vi "Transmit Reference (FPGA).vi"() -> ()   [LabVIEW 2019]
uses:
  SubVIs/Tone Generator/Channel Control.ctl
  SubVIs/Sync/Sync Control.ctl
  SubVIs/Sync/Sync Measurements.ctl
  <instrlib>/_niInstr/DSP/v1/Shared/Public/IQ Impairments.ctl
  <instrlib>/_niInstr/DSP/v1/Shared/Public/Filter Coefficients.ctl
  Host/SubVIs/Low-level/TypeDefs/Gain Setting.ctl
  <instrlib>/niMmWave/ni3620/Config/v1/FPGA/Public/Typedefs/TX1 RX1 Port.ctl
  <vilib>/Platform/TimedLoop/XDataNode/timing_clust.ctl
  <vilib>/Platform/TimedLoop/XDataNode/nitl_modes.ctl
  <vilib>/Platform/TimedLoop/XDataNode/wakeup.ctl
  <instrlib>/_niInstr/DSP/v1/Shared/Public/IQ Data.ctl
  <vilib>/rvi/Emulation/niFpgaSctlEmulationGetInTimedLoop.vi
  <vilib>/rvi/Emulation/niFpgaEmulationReportErrorSimple.vi
  <vilib>/rvi/Emulation/niFpgaGetClockAttributes.vi
  <vilib>/rvi/Emulation/niFpgaCriticalErrorInLSC.vi
  <vilib>/rvi/Emulation/niFpgaProcessEmulError.vi
  <vilib>/rvi/eio/common/nirviEmuTemplateMethod_errors.vi
  SubVIs/Misc/Globals.vi
  <vilib>/rvi/interface/RandomDataEmulation/nirviRandomDataMultiElementFPGAFIFO.vi
  <instcachedir>/0/nirviRandomDataMultiElementFPGAFIFO_1ED88BA00AC641F388A9B1FAA20E354D.lvgen/nirviRandomDataMultiElementFPGAFIFO_1ED88BA00AC641F388A9B1FAA20E354D_003.vi
  <vilib>/rvi/interface/RandomDataEmulation/niFpgaRandomDataHandleErrors.vi
  <instrlib>/_niInstr/Basic Elements/v1/FPGA/Private/Count Up U16.vi
  <instrlib>/_niInstr/Data Formatting/v1/FPGA/Private/Convert/U32 array to Boolean Array.vi
  <vilib>/rvi/Memory/Memory_Emulation/nirvimemoryFastEmulation.vi
  <vilib>/rvi/Memory/Memory_Emulation/nirvimemoryEmulation.vi
  <vilib>/rvi/Emulation/niFpgaEmulationIsFPGAContextNoSignature.vi
  <vilib>/rvi/DataTransferAndStorage/Container/Common/niFpgaContainerGetUniqueNameForEmu.vi
  <vilib>/rvi/errors/nirviReportUnexpectedCaseInternalError (U32).vi
  <instrlib>/_niInstr/Data Formatting/v1/FPGA/Private/Convert/U8 array to Boolean Array.vi
  <instrlib>/_niInstr/Data Formatting/v1/FPGA/Private/Convert/Boolean Array to U32 Array.vi
  <vilib>/rvi/errors/niFpgaSetErrorForExecOnDevCompSimple.vi
  <vilib>/rvi/eio/common/nirviEmuReportErrorAndStop.vi
  <vilib>/rvi/FIFO/Fifo_Resource/nirvififoEmulationSetSize.vi
  <vilib>/rvi/FIFO/Fifo_Resource/nirviFifoEmulationQueueMgr.vi
  <instcachedir>/0/nirviFifoEmulationQueueMgr_E5CAEC123FF24DC58D834DCA3CDAA9B5.lvgen/nirviFifoEmulationQueueMgr_E5CAEC123FF24DC58D834DCA3CDAA9B5_008.vi
  <vilib>/rvi/FIFO/Fifo_Resource/nirvififoEmulationDetermineInputValidOut.vi
  <vilib>/rvi/FIFO/Fifo_Resource/nirvififoEmulationCreateLock.vi
  <vilib>/rvi/FIFO/Fifo_Resource/nirvififoEmulationObtainLock.vi
  <vilib>/rvi/FIFO/Fifo_Resource/nirvififoEmulationReleaseLock.vi
  <vilib>/rvi/occurrence/nirviWaitOnOccurrenceBase.vi
  <vilib>/rvi/errors/nirviReportUnexpectedCaseInternalError.vi
  <instrlib>/_niInstr/Basic Elements/v1/FPGA/Private/Count Up U8.vi
  <vilib>/rvi/DataTransferAndStorage/Container/Common/niFpgaContainerSetEmuInfo.vi
  <vilib>/Utility/error.llb/Clear Errors.vi
  <vilib>/Platform/TimedLoop/XDataNode/XDataNode.xnode
  <vilib>/eio/EIONode/EIONode.xnode
  <vilib>/eio/EIOMethodNode/EIOMethodNode.xnode
  <vilib>/rvi/DataTransferAndStorage/Container/XNode/niFpgaContainer.xnode
  <vilib>/rvi/interface/RandomDataEmulation/nirviRandomDataFpgaMultiElementTemplate.vi
  <vilib>/rvi/FIFO/Fifo_Resource/nirvififoEmulationWrite.vi
  <vilib>/rvi/LocalResourceManager/LocalResourceManager.xnode
  <vilib>/rvi/FIFO/Fifo_Resource/nirvififoEmulationRead.vi
  <vilib>/Platform/TimedLoop/XDataNode/XDNodeRunTimeDep.lvlib
  <instrlib>/_niInstr/Basic Elements/v1/FPGA/niInstr Basic Elements v1 FPGA.lvlib
  <instrlib>/_niInstr/Data Formatting/v1/FPGA/niInstr Data Formatting v1 FPGA.lvlib
  <instrlib>/_niInstr/DSP/v1/Shared/niInstr DSP v1 Shared.lvlib
  <instrlib>/niMmWave/ni3620/Config/v1/FPGA/niMmWave Config v1 FPGA.lvlib
panel:
  in  "sync.master reset listen":bool
  in  "sync.counter reset enable":bool
  in  "20 kHz tclk parameters":T1
  out "sysref value":u8
  out "tclk value":u16
  in  "gain ranging.enable port config":bool
  in  "gain ranging.enable coarse gain ranging":bool
  in  "gain ranging.enable fine gain ranging":bool
  in  "gain ranging.coarse gain values":fxp<+/-,16,12>[](array[numeric])=[0.0, 0.0, 0.0, 0.0]
  out "port 5.debug info":T2
  out "port 5.rx fifo overflow":bool
  in  "port 5.rx fifo overflow clear":bool
  out "port 4.rx fifo overflow":bool
  in  "port 4.rx fifo overflow clear":bool
  out "port 4.debug info":T2
  out "aurora.fifo 1 overflow":bool
  in  "aurora.reset trigger":bool
  out "aurora.fifo 0 overflow":bool
  in  "aurora.fifo overflow clear":bool
  in  "aurora.write":bool
  out "clocks valid":bool[](array[boolean])
  in  "table info":T3
  in  "gain ranging.manual setting":T6
  in  "gain ranging.setting list step":T7
  in  "gain ranging.enable":bool
  in  "gain ranging.dwell time (cycles)":u32=4800
  in  "txjesd.control":T8
  out "txjesd.status":T9
  in  "filter.enable":bool
  in  "filter.coefficients":T10
  in  "cal.correction":T12={"sample delay"={"I delay"=0.0, "Q delay"=0.0}, "fractional delay"={"enable"=FALSE, "coef write"=FALSE, "coef data"=0.0}, "impairments"={"inline gain I"=0.9999923706054688, "inline gain Q"=0.9999923706054688, "cross gain I"=0.0, "cross gain Q"=0.0, "pre-gain offset I"=0.0, "pre-gain offset Q"=0.0, "post-gain offset I"=0.0, "post-gain offset Q"=0.0}, "iq inversion"={"invert I"=FALSE, "invert Q"=FALSE}}
  out "sync.measurements":T13
  in  "sync.parameters":T15
  in  "sync.use synced trigger":bool
  in  "sync.trigger":bool
  in  "gen.read":bool
  in  "cal.generation":T16={"generation select"=enum."Pass Through", "tone parameters"={"frequency"=0.125, "gain"=0.5}, "pulse parameters"={"frequency"=16, "gain"=0.5, "width"=16}}
  in  "gen.load":bool
  in  "gen.triggered read":bool
  in  "gen.length":u16=15
  in  "gen.write enable":bool
  in  "tone.routing":cluster{"I":T17, "Q":T17}
  in  "tone.parameters":T18(array[cluster])=[{"frequency"=0.032551999999999026, "gain"=0.8000030517578125, "phase"=0.0, "offset"={"offset I"=0.0, "offset Q"=0.0}}, {"frequency"=0.032551999999999026, "gain"=0.0, "phase"=0.0, "offset"={"offset I"=0.0, "offset Q"=0.0}}] {"offset"."offset Q" format="%#.18g"; "offset"."offset I" format="%#.18g"}
  in  "waveform type":enum16{"Tone", "Waveform Generation"}(ring)
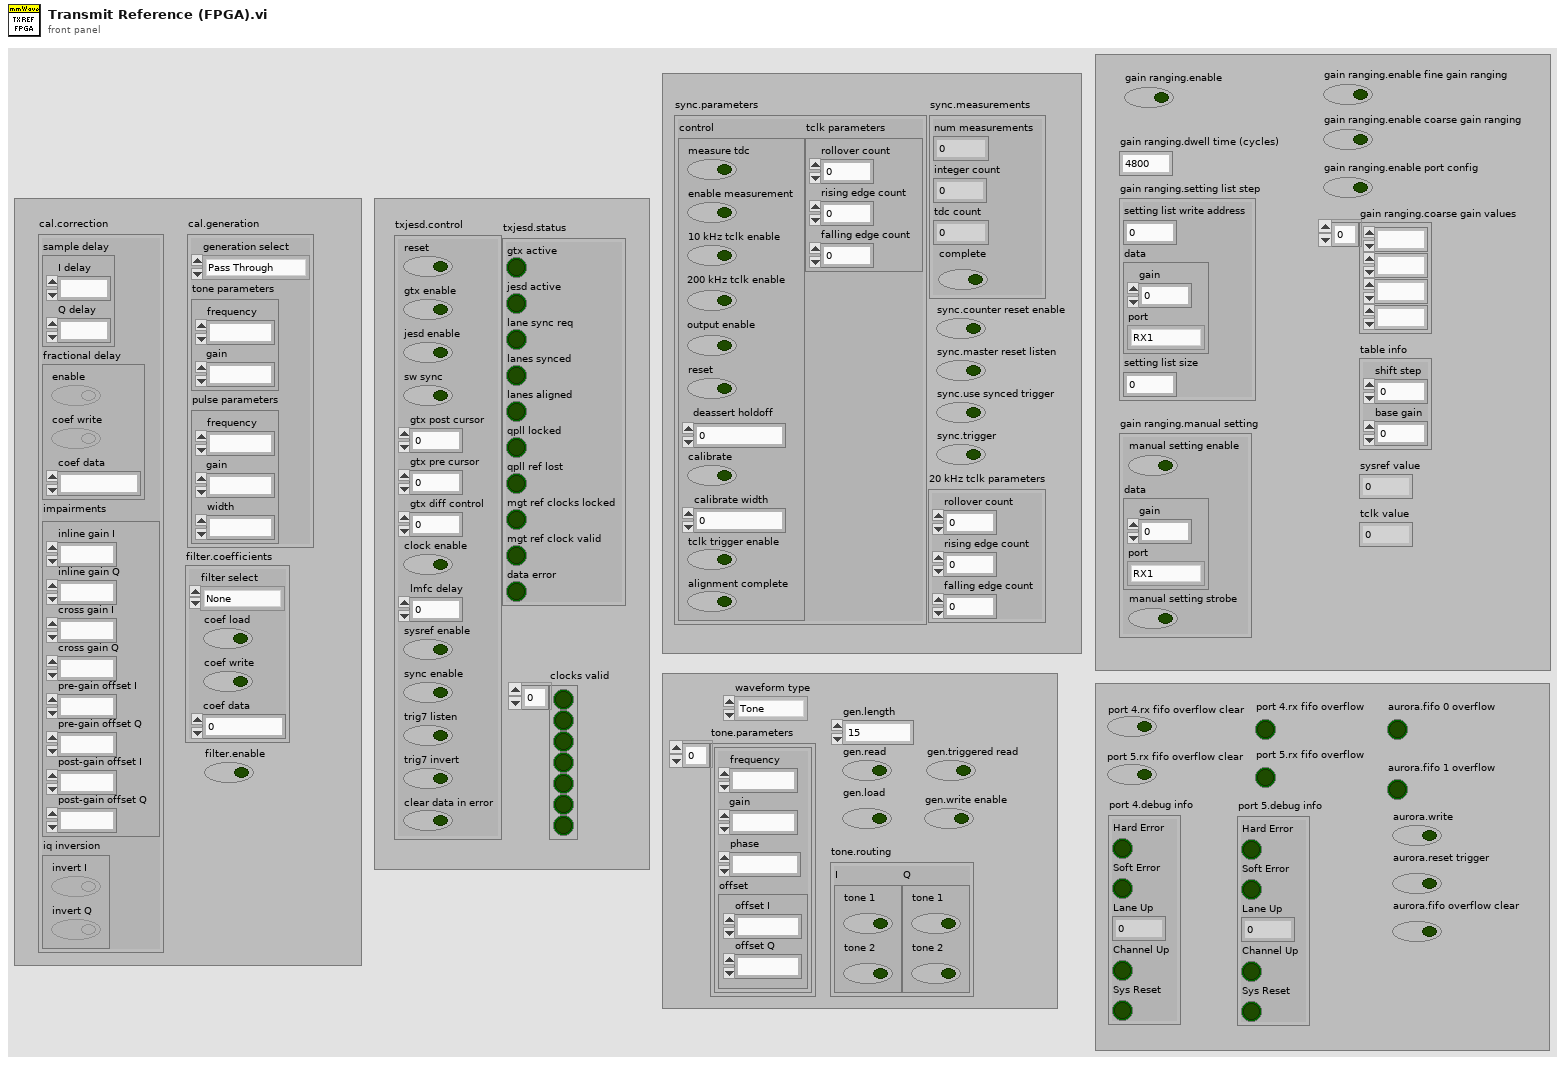
[diagram p1: front panel]
types:
  T1 = cluster{"rollover count":u16, "rising edge count":u16, "falling edge count":u16}
  T2 = cluster{"Hard Error":bool, "Soft Error":bool, "Lane Up":fxp<+,4,4>, "Channel Up":bool, "Sys Reset":bool}
  T3 = cluster{"shift step":i16, "base gain":fxp<+/-,16,12>}
  T4 = typedef "gain setting.ctl" = cluster{"gain":fxp<+/-,16,12>, "port":T5}
  T5 = typedef "TX1 RX1 Port.ctl" = enum8{"RX1", "TX1/RX2"}
  T6 = cluster{"manual setting enable":bool, "data":T4, "manual setting strobe":bool}
  T7 = cluster{"setting list write address":u32, "data":T4, "setting list size":u16}
  T8 = cluster{"reset":bool, "gtx enable":bool, "jesd enable":bool, "sw sync":bool, "gtx post cursor":fxp<+,5,5>, "gtx pre cursor":fxp<+,5,5>, "gtx diff control":fxp<+,4,4>, "clock enable":bool, "lmfc delay":fxp<+,5,5>, "sysref enable":bool, "sync enable":bool, "trig7 listen":bool, "trig7 invert":bool, "clear data in error":bool}
  T9 = cluster{"gtx active":bool, "jesd active":bool, "lane sync req":bool, "lanes synced":bool, "lanes aligned":bool, "qpll locked":bool, "qpll ref lost":bool, "mgt ref clocks locked":bool, "mgt ref clock valid":bool, "data error":bool}
  T10 = typedef "niInstr DSP v1 Shared.lvlib/Filter Coefficients.ctl" = cluster{"filter select":enum8{"None", "I Inline", "I Cross", "Q Cross", "Q Inline"}, "coef load":bool, "coef write":bool, "coef data":fxp<+/-,18,1>}
  T11 = typedef "niInstr DSP v1 Shared.lvlib/IQ Impairments.ctl" = cluster{"inline gain I":fxp<+/-,18,1>, "inline gain Q":fxp<+/-,18,1>, "cross gain I":fxp<+/-,18,1>, "cross gain Q":fxp<+/-,18,1>, "pre-gain offset I":fxp<+/-,18,1>, "pre-gain offset Q":fxp<+/-,18,1>, "post-gain offset I":fxp<+/-,18,1>, "post-gain offset Q":fxp<+/-,18,1>}
  T12 = cluster{"sample delay":cluster{"I delay":fxp<+,13,13>, "Q delay":fxp<+,13,13>}, "fractional delay":cluster{"enable":bool, "coef write":bool, "coef data":fxp<+/-,18,1>}, "impairments":T11, "iq inversion":cluster{"invert I":bool, "invert Q":bool}}
  T13 = typedef "Sync Measurements.ctl" = cluster{"num measurements":u16, "integer count":u16, "tdc count":u16, "complete":bool}
  T14 = typedef "Sync Control.ctl" = cluster{"measure tdc":bool, "enable measurement":bool, "10 kHz tclk enable":bool, "200 kHz tclk enable":bool, "output enable":bool, "reset":bool, "deassert holdoff":u8, "calibrate":bool, "calibrate width":u8, "tclk trigger enable":bool, "alignment complete":bool}
  T15 = cluster{"control":T14, "tclk parameters":cluster{"rollover count":u16, "rising edge count":u16, "falling edge count":u16}}
  T16 = cluster{"generation select":enum16{"Pass Through", "Tone", "Pulse", "Disable"}, "tone parameters":cluster{"frequency":fxp<+/-,48,0>, "gain":fxp<+/-,18,1>}, "pulse parameters":cluster{"frequency":u32, "gain":fxp<+/-,18,1>, "width":u8}}
  T17 = typedef "Channel Control.ctl" = cluster{"tone 1":bool, "tone 2":bool}
  T18 = cluster{"frequency":fxp<+/-,48,0>, "gain":fxp<+/-,18,1>, "phase":fxp<+/-,21,0>, "offset":cluster{"offset I":fxp<+/-,18,1>, "offset Q":fxp<+/-,18,1>}}[]
  T19 = cluster{"s_axis_tvalid":refnum<k21>, "s_axis_tdata_0":refnum<k21>, "s_axis_tdata_1":refnum<k21>, "s_axis_tdata_2":refnum<k21>, "s_axis_tdata_3":refnum<k21>, "s_axis_tready":refnum<k21>}
  T20 = cluster{"m_axis_tvalid":refnum<k21>, "m_axis_tdata_0":refnum<k21>, "m_axis_tdata_1":refnum<k21>, "m_axis_tdata_2":refnum<k21>, "m_axis_tdata_3":refnum<k21>}
  T21 = typedef "Sync Resources.ctl" = cluster{"tdc assert":refnum<k21>, "tdc deassert":refnum<k21>, "tdc count":refnum<k21>, "control":refnum<k21>, "integer count":refnum<k21>}
  T22 = typedef "XDNodeRunTimeDep.lvlib/timing_clust.ctl" = cluster{"Expected End [f-1]":u64, "Actual End [f-1]":u64, "Finished Late? [f-1]":bool, "Expected End [i-1]":u64, "Actual End [i-1]":u64, "Finished Late? [i-1]":bool, "Expected Start [i]":u64, "Actual Start [i]":u64, "Expected Start [f]":u64, "Actual Start [f]":u64, "Source Name":string, "Structure Name":string, "Period":i64, "Deadline":i64, "Offset":i64, "Start":i64, "Priority":i32, "Timeout":i32, "Mode":T23, "Wakeup Reason":T24, "Error":errorcluster, "Source Type":string, "Secondary Source Type":string, "Global End Time":u64, "Global Start Time":u64, "Frame Duration":u64, "Iteration Duration":u64, "Assigned CPU":i32, "I/O Scan Engine Mode":u32}
  T23 = typedef "XDNodeRunTimeDep.lvlib/nitl_modes.ctl" = enum32{"No Change", "Process missed periods, maintain original phase", "Discard missed periods, maintain original phase", "Process missed periods, ignore original phase", "Discard missed periods, ignore original phase"}
  T24 = typedef "XDNodeRunTimeDep.lvlib/wakeup.ctl" = enum32{"Normal", "Aborted", "Asynchronous wakeup", "Timing source error", "Timed loop error", "Timeout"}
  T25 = typedef "AXI4-Stream Reader FXP64x4 Resources.ctl" = cluster{"AXI4-Stream Reader Resources":cluster{"Use TREADY":bool, "Use TLAST":bool, "TLAST":refnum<k21>, "TREADY":refnum<k21>, "TVALID":refnum<k21>, "Use TKEEP":bool, "Use TSTRB":bool, "Use TUSER":bool}, "TDATA Resources":cluster{"TDATA_0":refnum<k21>, "TDATA_1":refnum<k21>, "TDATA_2":refnum<k21>, "TDATA_3":refnum<k21>}, "TKEEP":refnum<k21>, "TSTRB":refnum<k21>}
  T26 = typedef "AXI4-Stream Writer FXP64x4 Resources.ctl" = cluster{"Writer Resources":cluster{"Use TREADY":bool, "Use TLAST":bool, "TLAST":refnum<k21>, "TREADY":refnum<k21>, "TVALID":refnum<k21>, "Use TSTRB":bool, "Use TKEEP":bool, "Use TUSER":bool}, "TDATA Resources":cluster{"TDATA_0":refnum<k21>, "TDATA_1":refnum<k21>, "TDATA_2":refnum<k21>, "TDATA_3":refnum<k21>}, "TKEEP":refnum<k21>, "TSTRB":refnum<k21>}
  T27 = cluster{"disable TClk measure":bool, "output enable":bool, "output value":bool}
  T28 = typedef "niInstr DSP v1 Shared.lvlib/IQ Data.ctl" = cluster{"I":fxp<+/-,18,1>, "Q":fxp<+/-,18,1>, "overflow":bool}
  T29 = cluster{"Hard Error":refnum<k21>, "Soft Error":refnum<k21>, "Lane Up":refnum<k21>, "Channel Up":refnum<k21>, "Sys Reset":refnum<k21>}
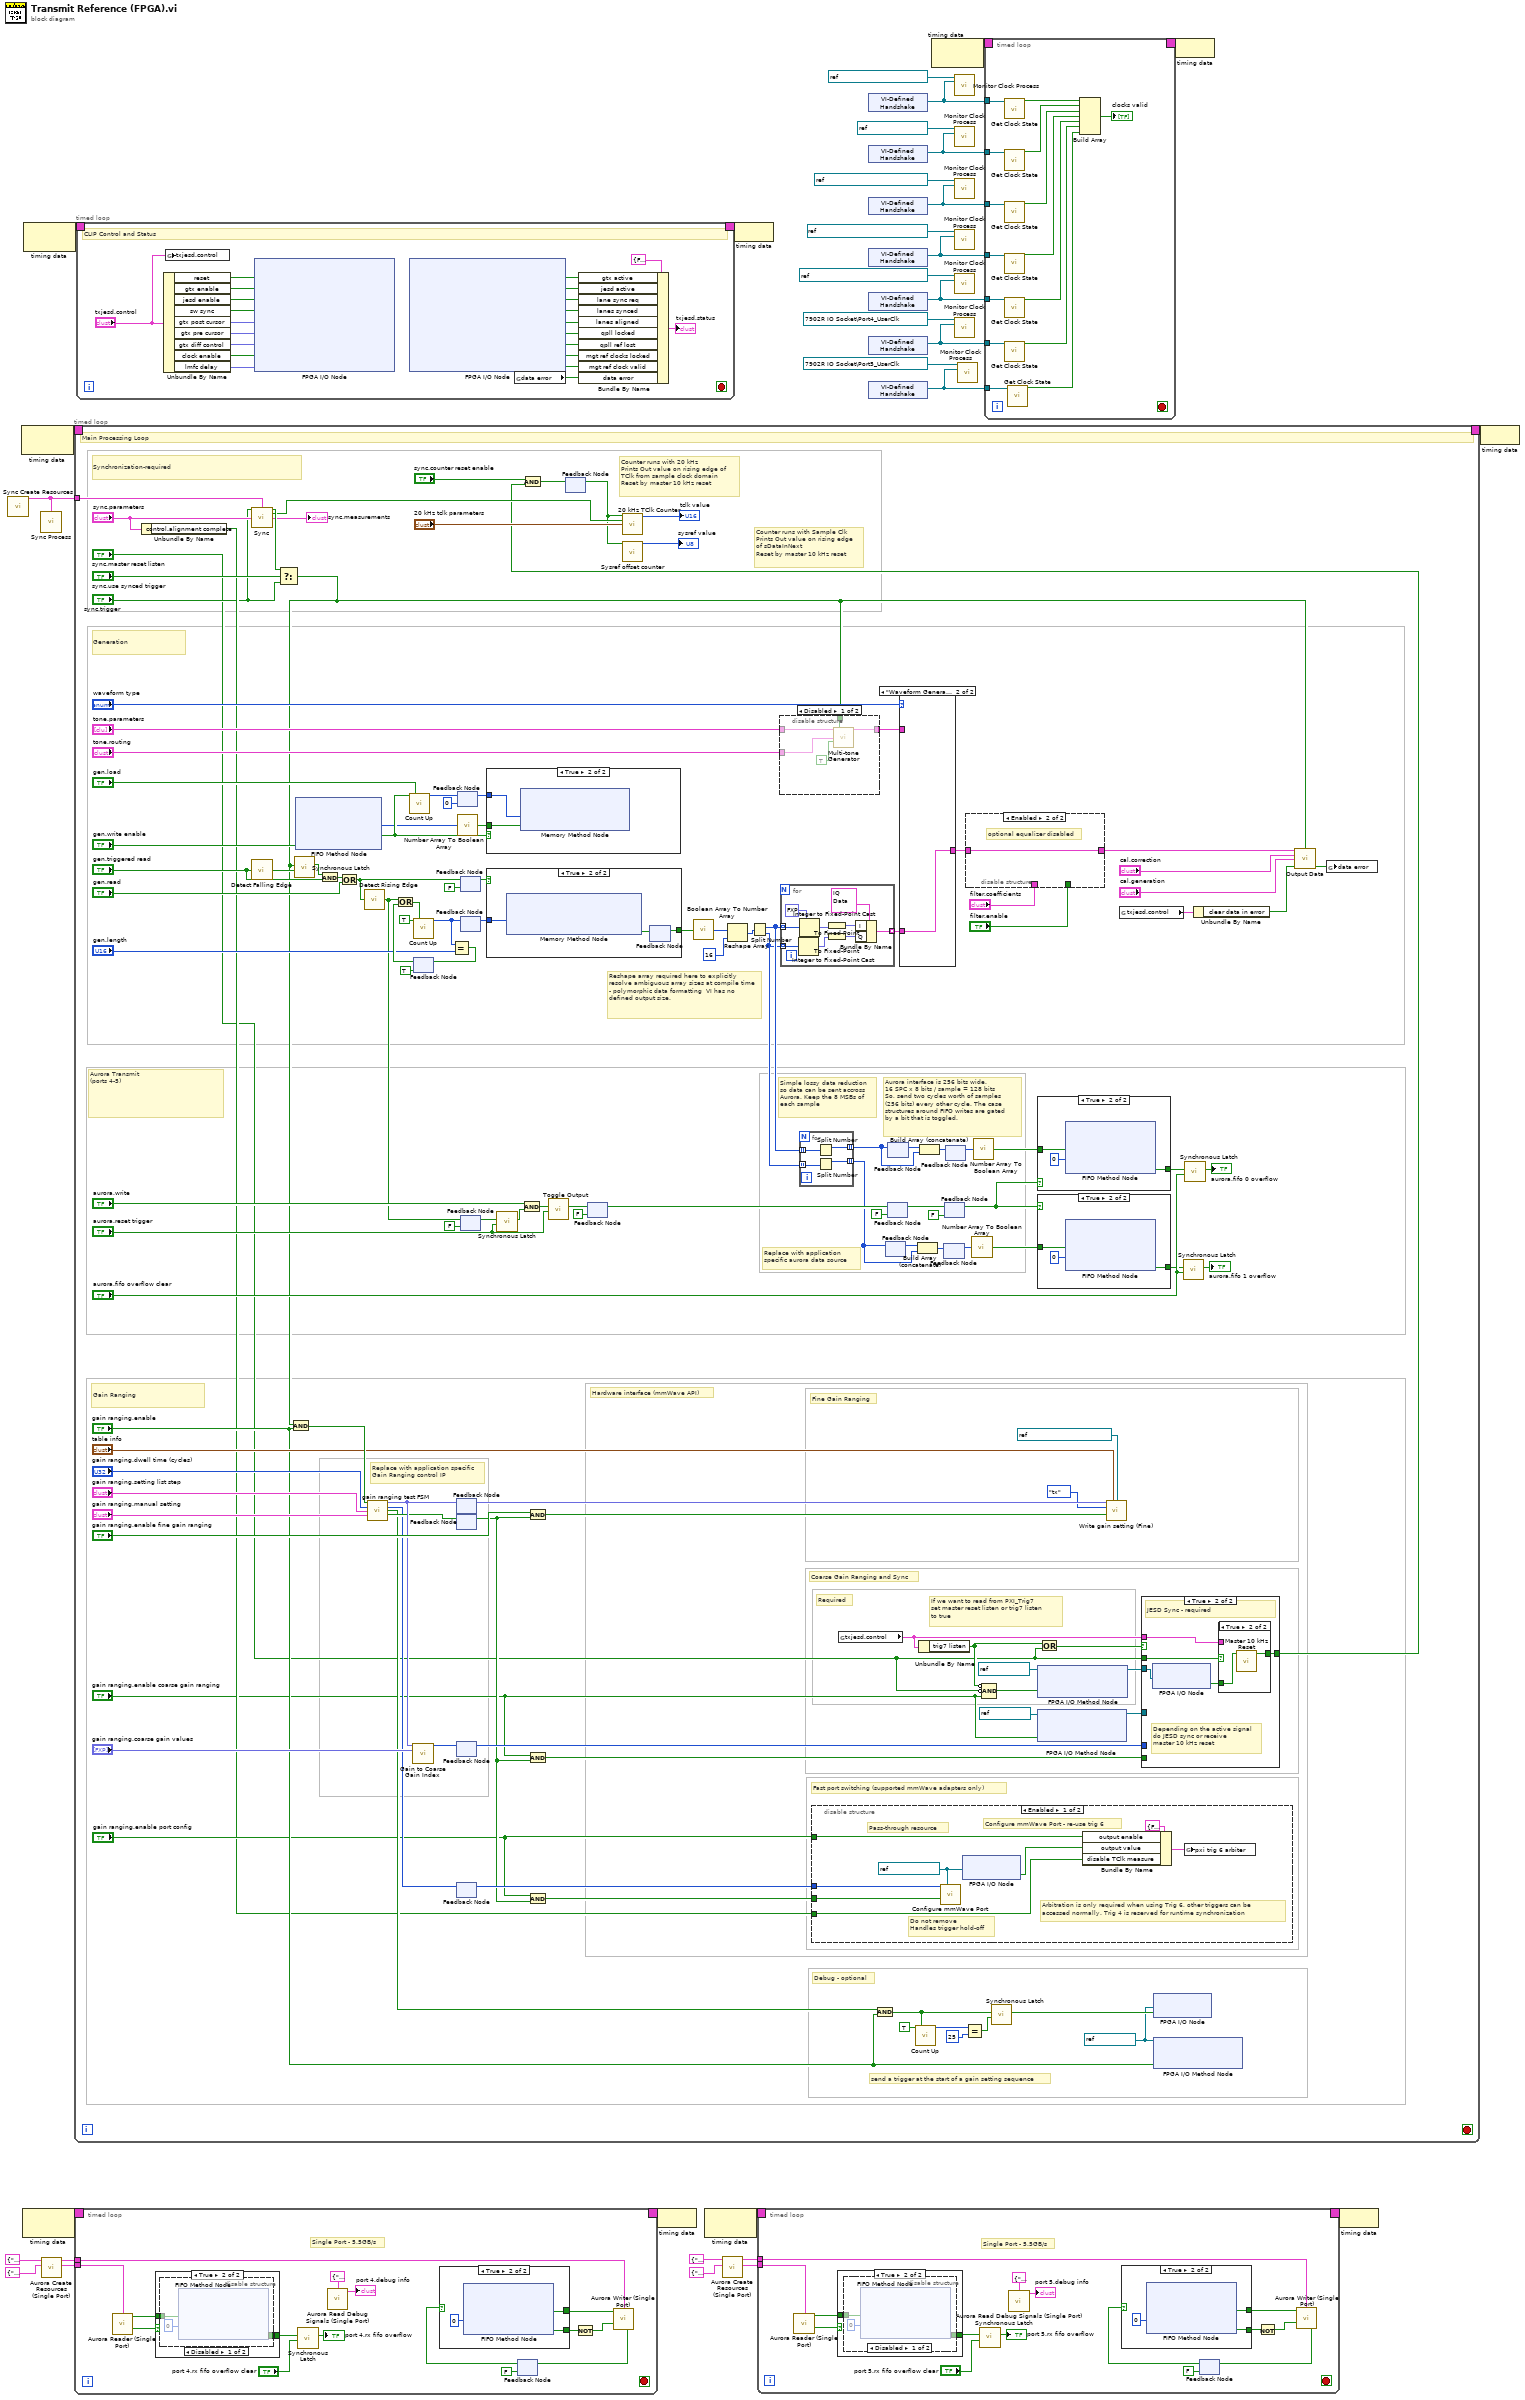
[diagram p0: block diagram]
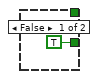
[diagram p2: hidden frame]
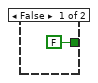
[diagram p3: hidden frame]
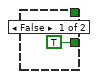
[diagram p5: hidden frame]
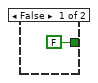
[diagram p6: hidden frame]
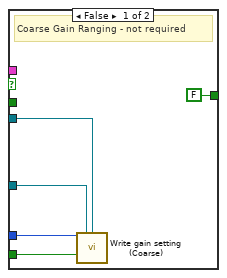
[diagram p9: hidden frame]
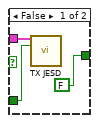
[diagram p10: hidden frame]
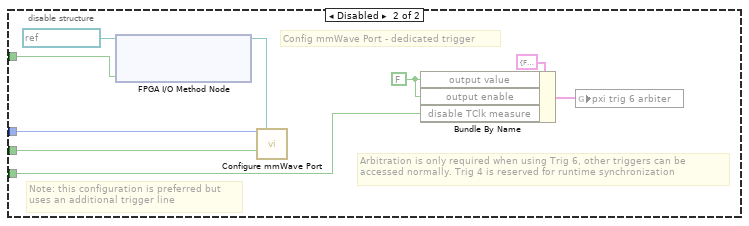
[diagram p11: hidden frame]
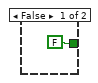
[diagram p12: hidden frame]
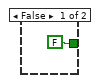
[diagram p13: hidden frame]
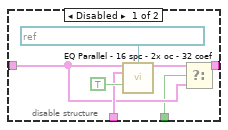
[diagram p14: hidden frame]
diagram:
  n1 = call "Sync Create Resources.vi"() -> ("sync.resources"=w29:T21)  [unwired: 15 in]
  n2 = node-c288() -> (w31:T22)  [unwired: 1 in]
  n3 = node-c288() -> (w12:T22)  [unwired: 1 in]
  n4 = node-c288() -> (w33:T22)  [unwired: 1 in]
  n5 = call "Sync Process.vi"("sync.resources"=w29) -> ()  [unwired: 15 in]
  n6 = call "Aurora Create Resources (Single Port).vi"("RX CLIP Resources"=T20 {"m_axis_tvalid"="7902R IO Socket\\uPort4_m_axi_rx_tvalid", "m_axis_tdata_0"="7902R IO Socket\\uPort4_m_axi_rx_tdata_0", "m_axis_tdata_1"="7902R IO Socket\\uPort4_m_axi_rx_tdata_1", "m_axis_tdata_2"="7902R IO Socket\\uPort4_m_axi_rx_tdata_2", "m_axis_tdata_3"="7902R IO Socket\\uPort4_m_axi_rx_tdata_3"}, "TX CLIP Resources"=T19 {"s_axis_tvalid"="7902R IO Socket\\uPort4_s_axi_tx_tvalid", "s_axis_tdata_0"="7902R IO Socket\\uPort4_s_axi_tx_tdata_0", "s_axis_tdata_1"="7902R IO Socket\\uPort4_s_axi_tx_tdata_1", "s_axis_tdata_2"="7902R IO Socket\\uPort4_s_axi_tx_tdata_2", "s_axis_tdata_3"="7902R IO Socket\\uPort4_s_axi_tx_tdata_3", "s_axis_tready"="7902R IO Socket\\uPort4_s_axi_tx_tready"}) -> ("AXI4-Stream Reader FXP64x4"=w8:T25, "AXI4-Stream Writer FXP64x4"=w7:T26)  [unwired: 8 in]
  n7 = timed-loop {
    timing: w31 -> [_]
    timing-out: [_] -> w30
    tunnel: w29 -> [w47]
    stop <- _ stop-if-true
    w65 = refnum<k21> "PXI_Trig3" ("FPGA I/O In")
    # "Counter runs with Sample Clk\nPrints Out value on rising edge\nof sDataInNext\nReset by master 10 kHz reset"
    # "If we want to read from PXI_Trig7\nset master reset listen or trig7 listen\nto true"
    # "Counter runs with 20 kHz\nPrints Out value on rising edge of \nTClk from sample clock domain\nReset by master 10 kHz reset"
    # "Aurora interface is 256 bits wide.\n16 SPC x 8 bits / sample = 128 bits\nSo, send two cycles worth of samples\n(256 bits) every other cycle. The case\nstructures around FIFO writes are gated\nby a bit that is toggled."
    # "Simple lossy data reduction\nso data can be sent accross\nAurora. Keep the 8 MSBs of\neach sample"
    # "Replace with application \nspecific aurora data source"
    # "Replace with application specific Gain Ranging control IP"
    # "Fast port switching (supported mmWave adapters only)"
    # "Fine Gain Ranging"
    # "Gain Ranging"
    # "Synchronization-required"
    # "Aurora Transmit\n(ports 4-5)"
    # "Hardware interface (mmWave API)"
    # "Generation"
    # "Coarse Gain Ranging and Sync"
    # "Debug - optional"
    # "Required"
    # "Required"
    # "send a trigger at the start of a gain setting sequence"
    # "Reshape array required here to explicitly resolve ambiguous array sizes at compile time - polymorphic data formatting  VI has no defined output size."
    # "Main Processing Loop"
    n8 = Unbundle By Name("sync.parameters") -> ("control.alignment complete"=w50:bool)
    n9 = call "Sync.vi"("trigger"="sync.trigger", "sync.resources"=w47, "sync.parameters"="sync.parameters") -> ("synced trigger"=w136:bool, "tclk"=w49:bool, "sync measurements"=→"sync.measurements":T13)  [unwired: 10 in]
    n10 = call <instrlib>:"Detect Falling Edge.vi"("signal"="gen.triggered read") -> ("edge detected"=w140:bool)  [unwired: 14 in]
    n11 = Select(t=w136, s="sync.use synced trigger", f="sync.trigger") -> (s? t:f=w35:bool)
    n12 = And(x=w35, y="gain ranging.enable") -> (x .and. y?=w120:bool)
    n13 = call <instrlib>:"Synchronous Latch.vi"("clear"=w140, "set"=w35) -> ("out"=w142:bool)  [unwired: 9 in]
    n14 = xnode ("FIFO Method Node")("Ready for Output"="gen.write enable") -> ("Element"=w137:u32[], "Output Valid"=w146:bool)  [unwired: 1 in, 1 out]
    n15 = And(x=w142, y="gen.triggered read") -> (x .and. y?=w139:bool)
    n16 = Or(x=w139, y="gen.read") -> (x .or. y?=w127:bool)
    n17 = call <instrlib>:"Detect Rising Edge.vi"("signal"=w127) -> ("edge detected"=w98:bool)  [unwired: 14 in]
    n18 = call "gain ranging test FSM.vi"("gain ranging.start sequence"=w120, "gain ranging.dwell time (cycles)"="gain ranging.dwell time (cycles)", "gain ranging.gain setting list"="gain ranging.setting list step", "gain ranging.manual request"="gain ranging.manual setting") -> ("gain ranging.gain setting"=w77:fxp<+/-,16,12>, "gain ranging.TX1/RX1 Port Value"=w74:T5, "gain ranging.start of sequence"=w64:bool, "gain ranging.gain setting valid"=w75:bool)  [unwired: 8 in]
    n19 = call-poly <instrlib>:"Count Up.vi"("increment"=w146, "reset"="gen.load") -> ("count out"=w149:u16)  [unwired: 13 in]
    n20 = call "Gain to Coarse Gain Index.vi"("gain setting"=w77, "coarse gain values"="gain ranging.coarse gain values") -> ("coarse gain index"=w81:u32)  [unwired: 13 in]
    n21 = feedback #1(TRUE) -> (w126:bool)
    n22 = Or(x=w98, y=w126) -> (x .or. y?=w125:bool)
    n23 = call-poly <instrlib>:"Count Up.vi"("increment"=TRUE, "reset"=w125) -> ("count out"=w124:u16)  [unwired: 13 in]
    n24 = Equal?(x=w124, y="gen.length") -> (x = y?=w154:bool)
    n25 = feedback-in #1(w154) -> ()
    n26 = feedback #2() -> (w79:fxp<+/-,16,12>)  [unwired: 1 in]
    n27 = feedback-in #2(w77) -> ()
    n28 = feedback #3() -> (w53:bool)  [unwired: 1 in]
    n29 = feedback-in #3(w75) -> ()
    n30 = feedback #4() -> (w63:u32)  [unwired: 1 in]
    n31 = feedback-in #4(w81) -> ()
    n32 = feedback #5() -> (w73:T5)  [unwired: 1 in]
    n33 = feedback-in #5(w74) -> ()
    n34 = feedback-in #6(w149) -> ()
    n35 = feedback #6(u16 0 ("count out")) -> (w148:u16)
    n36 = call-poly <instrlib>:"Number Array To Boolean Array.vi"("data in"=w137) -> ("data out"=w159:bool[])  [unwired: 14 in]
    n37 = feedback #7(FALSE ("gen mem.read")) -> (w157:bool)
    n38 = feedback-in #7(w127) -> ()
    n39 = feedback #8() -> (w158:u16)  [unwired: 1 in]
    n40 = feedback-in #8(w124) -> ()
    n41 = feedback #9(FALSE ("edge detected")) -> (w97:bool)
    n42 = feedback-in #9(w98) -> ()
    n43 = case shown="True" w146 {
      tunnel: w159 -> [_ w233]
      tunnel: w148 -> [_ w232]
      frame False {
      }
      frame True {
        n44 = xnode ("Memory Method Node")("Address"=w232, "Data"=w233) -> ()  [unwired: 1 in, 1 out]
      }
    }
    n45 = case shown="True" w157 {
      tunnel: w158 -> [_ w220]
      tunnel: [_ w221] -> w155
      frame False {
      }
      frame True {
        n46 = xnode ("Memory Method Node")("Address"=w220) -> ("Data"=w222:bool[])  [unwired: 1 in, 1 out]
        n47 = feedback #10() -> (w221:bool[])  [unwired: 1 in]
        n48 = feedback-in #10(w222) -> ()
      }
    }
    n49 = call <instrlib>:"Synchronous Latch.vi"("clear"="aurora.reset trigger", "set"=w97) -> ("out"=w102:bool)  [unwired: 9 in]
    n50 = And(x="aurora.write", y=w102) -> (x .and. y?=w110:bool)
    n51 = And(x="gain ranging.enable fine gain ranging", y=w53) -> (x .and. y?=w78:bool)
    n52 = And(x="gain ranging.enable coarse gain ranging", y=w53) -> (x .and. y?=w62:bool)
    n53 = And(x="gain ranging.enable port config", y=w53) -> (x .and. y?=w54:bool)
    n54 = call <instrlib>:"Toggle Output.vi"("clear"="aurora.reset trigger", "toggle"=w110) -> ("output"=w90:bool)  [unwired: 9 in]
    n55 = feedback #11() -> (w36:bool)  [unwired: 1 in]
    n56 = feedback #12(FALSE) -> (w86:bool)
    n57 = feedback-in #12(w90) -> ()
    n58 = call "20 kHz TClk Counter.vi"("master 10 kHz reset"=w36, "tclk"=w49, "20 kHz tclk parameters"="20 kHz tclk parameters") -> ("tclk offset value"=→"tclk value":u16)  [unwired: 12 in]
    n59 = call "Sysref offset counter.vi"("master 10 kHz reset"=w36) -> ("sysref offset value"=→"sysref value":u8)  [unwired: 14 in]
    n60 = call-poly <instrlib>:"Boolean Array To Number Array.vi"("data in"=w155) -> ("data out"=w96:u32[])  [unwired: 14 in]
    n61 = Reshape Array(w96, 16 ("dimension size")) -> (w94:u32[])
    n62 = Split Number(x=w94) -> (hi(x)=w93:u16[], lo(x)=w92:u16[])
    n63 = disable-structure shown="Disabled" {
      disable-tunnel: "tone.parameters" -> [w167 _]
      disable-tunnel: "tone.routing" -> [w166 _]
      disable-tunnel: [w165 _] -> w144
      disable-tunnel: w35 -> [w163 _]
      frame Disabled {
        n64 = call "Multi-tone Generator.vi"("tone.parameters"=w167, "tone.reset"=w163, "tone routing"=w166, "input valid"=TRUE) -> ("tone data"=w165:T28[])  [unwired: 10 in, 1 out]
      }
      frame Enabled {
      }
    }
    n65 = for {
      tunnel: [w229] -> w151 mode=indexing
      tunnel: w93 -> [w228] mode=indexing
      tunnel: w92 -> [w227] mode=indexing
      w224 = fxp<+/-,16,1> 0.0 ("fixed-point type")
      n66 = Integer to Fixed-Point Cast(fixed-point type=w224, integer=w227) -> (fixed-point=w226:fxp<+/-,16,1>)
      n67 = Integer to Fixed-Point Cast(fixed-point type=w224, integer=w228) -> (fixed-point=w225:fxp<+/-,16,1>)
      n68 = To Fixed-Point(number=w225) -> (fixed-point=w231:fxp<+/-,18,1>)  [unwired: 1 in]
      n69 = To Fixed-Point(number=w226) -> (fixed-point=w230:fxp<+/-,18,1>)  [unwired: 1 in]
      n70 = Bundle By Name(cluster=T28 {"I"=0.0, "Q"=0.0, "overflow"=FALSE} ("data"), "I"=w231, "Q"=w230) -> (w229:T28)
    }
    n71 = for {
      tunnel: [w202] -> w112 mode=indexing
      tunnel: [w201] -> w85 mode=indexing
      tunnel: w93 -> [w203] mode=indexing
      tunnel: w92 -> [w200] mode=indexing
      n72 = Split Number(x=w203) -> (hi(x)=w202:u8)  [unwired: 1 out]
      n73 = Split Number(x=w200) -> (hi(x)=w201:u8)  [unwired: 1 out]
    }
    n74 = disable-structure shown="Enabled" {
      disable-tunnel: w54 -> [w188 w197]
      disable-tunnel: w73 -> [w187 w196]
      disable-tunnel: "gain ranging.enable port config" -> [w184 w192]
      disable-tunnel: w50 -> [w183 w191]
      frame Enabled {
        w186 = refnum<k21> "PXIe_DStarC" ("FPGA I/O In")
        # "Do not remove\nHandles trigger hold-off"
        # "Configure mmWave Port - re-use trig 6"
        # "Pass-through resource"
        # "Arbitration is only required when using Trig 6, other triggers can be accessed normally. Trig 4 is reserved for runtime synchronization"
        n75 = call <instrlib>:"Configure mmWave Port.vi"("port"=w187, "pxi trigger"=w186, "input valid"=w188) -> ()  [unwired: 12 in, 1 out]
        n76 = xnode "FPGA I/O Node"("FPGA I/O In"=w186) -> ("I/O Item"=w185:bool)  [unwired: 1 out]
        n77 = Bundle By Name(cluster=T27 {"disable TClk measure"=FALSE, "output enable"=FALSE, "output value"=FALSE} ("pxi trig 6 arbiter"), "output enable"=w184, "output value"=w185, "disable TClk measure"=w183) -> (w189:T27)
        n78 = global write "Globals.vi" "pxi trig 6 arbiter"(w189) -> ()
      }
      frame Disabled {
        w195 = FALSE ("disable TClk measure")
        # "Note: this configuration is preferred but \nuses an additional trigger line"
        # "Config mmWave Port - dedicated trigger"
        # "Arbitration is only required when using Trig 6, other triggers can be accessed normally. Trig 4 is reserved for runtime synchronization"
        n79 = xnode "FPGA I/O Method Node"("FPGA I/O In"=refnum<k21> "PXI_Trig0" ("pxi trigger 1"), "Enable"=w192) -> ("FPGA I/O Out"=w194:refnum<k21>)
        n80 = call <instrlib>:"Configure mmWave Port.vi"("port"=w196, "pxi trigger"=w194, "input valid"=w197) -> ()  [unwired: 12 in, 1 out]
        n81 = Bundle By Name(cluster=T27 {"disable TClk measure"=FALSE, "output enable"=FALSE, "output value"=FALSE} ("pxi trig 6 arbiter"), "output value"=w195, "output enable"=w195, "disable TClk measure"=w191) -> (w198:T27)
        n82 = global write "Globals.vi" "pxi trig 6 arbiter"(w198) -> ()
      }
    }
    n83 = global read "Globals.vi" "txjesd.control"() -> (w59:T8)
    n84 = And(x=w64, y="gain ranging.enable") -> (x .and. y?=w66:bool)
    n85 = feedback #13() -> (w106:u8[])  [unwired: 1 in]
    n86 = feedback-in #13(w85) -> ()
    n87 = feedback #14(FALSE) -> (w84:bool)
    n88 = feedback-in #14(w86) -> ()
    n89 = feedback #15() -> (w108:u8[])  [unwired: 1 in]
    n90 = feedback-in #15(w112) -> ()
    n91 = case shown="\"Waveform Generation\"" "waveform type" {
      tunnel: w144 -> [w234 _]
      tunnel: [w234 w235] -> w132
      tunnel: w151 -> [_ w235]
      frame "Tone", Default {
      }
      frame "Waveform Generation" {
      }
    }
    n92 = call-poly <instrlib>:"Count Up.vi"("increment"=TRUE, "reset"=w66) -> ("count out"=w70:u8)  [unwired: 13 in]
    n93 = Build Array (concatenate)(w106, w85) -> (w107:u8[])
    n94 = Unbundle By Name(w59) -> ("trig7 listen"=w40:bool)
    n95 = Build Array (concatenate)(w108, w112) -> (w109:u8[])
    n96 = feedback #16() -> (w116:u8[])  [unwired: 1 in]
    n97 = feedback-in #16(w107) -> ()
    n98 = feedback #17(FALSE) -> (w83:bool)
    n99 = feedback-in #17(w84) -> ()
    n100 = feedback #18() -> (w115:u8[])  [unwired: 1 in]
    n101 = feedback-in #18(w109) -> ()
    n102 = Equal?(x=w70, y=u8 25) -> (x = y?=w68:bool)
    n103 = disable-structure shown="Enabled" {
      disable-tunnel: "filter.coefficients" -> [w216 _]
      disable-tunnel: w132 -> [w214 w219]
      disable-tunnel: [w213 w219] -> w56
      disable-tunnel: "filter.enable" -> [w212 _]
      frame Disabled {
        n104 = call "EQ Parallel - 16 spc - 2x oc - 32 coef.vi"("data in"=w214, "clock x2"=refnum<k21> "7902R IO Socket\\SampleClkx2", "filter coefficients"=w216, "input valid"=TRUE) -> ("data out"=w215:T28[])  [unwired: 9 in, 2 out]
        n105 = Select(t=w215, s=w212, f=w214) -> (s? t:f=w213:T28[])
      }
      frame Enabled {
        # "optional equalizer disabled"
      }
    }
    n106 = call-poly <instrlib>:"Number Array To Boolean Array.vi"("data in"=w116) -> ("data out"=w114:bool[])  [unwired: 14 in]
    n107 = call-poly <instrlib>:"Number Array To Boolean Array.vi"("data in"=w115) -> ("data out"=w113:bool[])  [unwired: 14 in]
    n108 = Compound Arithmetic op=AND(invert w40, invert "sync.master reset listen", "gain ranging.enable coarse gain ranging") -> (w58:bool)
    n109 = call <instrlib>:"Synchronous Latch.vi"("clear"=w68, "set"=w66) -> ("out"=w67:bool)  [unwired: 9 in]
    n110 = xnode "FPGA I/O Method Node"("FPGA I/O In"=refnum<k21> "PXI_Trig5" ("pxi trigger 1"), "Enable"="gain ranging.enable coarse gain ranging") -> ("FPGA I/O Out"=w61:refnum<k21>)
    n111 = case shown="True" w83 {
      tunnel: [FALSE ("Timed Out?") w211] -> w100
      tunnel: w113 -> [_ w210]
      frame False {
      }
      frame True {
        n112 = xnode ("FIFO Method Node")("Element"=w210, "Timeout"=0) -> ("Timed Out?"=w211:bool)  [unwired: 1 in, 1 out]
      }
    }
    n113 = case shown="True" w83 {
      tunnel: [FALSE ("Timed Out?") w207] -> w104
      tunnel: w114 -> [_ w206]
      frame False {
      }
      frame True {
        n114 = xnode ("FIFO Method Node")("Element"=w206, "Timeout"=0) -> ("Timed Out?"=w207:bool)  [unwired: 1 in, 1 out]
      }
    }
    n115 = xnode "FPGA I/O Method Node"("FPGA I/O In"=refnum<k21> "PXI_Trig7" ("pxi trigger 1"), "Enable"=w58) -> ("FPGA I/O Out"=w60:refnum<k21>)
    n116 = Or(x=w40, y="sync.master reset listen") -> (x .or. y?=w44:bool)
    n117 = call <instrlib>:"Write gain setting (Fine).vi"("gain"=w79, "table info"="table info", "P2P Writer FIFO"=refnum<k21> "P2P FIFO to PXIe-3620" ("FIFO In"), "direction"=enum8{"rx", "tx"}."tx", "input valid"=w78) -> ()  [unwired: 10 in, 1 out]
    n118 = global read "Globals.vi" "txjesd.control"() -> (w129:T8)
    n119 = case shown="True" w44 {
      tunnel: w60 -> [w172 w175]
      tunnel: w61 -> [w171 _]
      tunnel: w63 -> [w170 _]
      tunnel: w62 -> [w169 _]
      tunnel: w59 -> [_ w176]
      tunnel: "sync.master reset listen" -> [_ w174]
      tunnel: [FALSE ("Master10k_Reset") w173] -> w39
      frame False {
        # "Coarse Gain Ranging - not required"
        n120 = call <instrlib>:"Write gain setting (Coarse).vi"("fast jump table index"=w170, "pxi trigger 1"=w171, "pxi trigger 2"=w172, "input valid"=w169) -> ()  [unwired: 11 in, 1 out]
      }
      frame True {
        # "Depending on the active signal\ndo JESD sync or receive\nmaster 10 kHz reset"
        # "JESD Sync - required"
        n121 = xnode "FPGA I/O Node"("FPGA I/O In"=w175) -> ("I/O Item"=w177:bool)  [unwired: 1 out]
        n122 = case shown="True" w174 {
          tunnel: w177 -> [w180 w182]
          tunnel: w176 -> [w179 _]
          tunnel: [FALSE ("Master10k_Reset") w181] -> w173
          frame False {
            n123 = call "TX JESD.vi"("txjesd.control"=w179, "trigger value"=w180) -> ()  [unwired: 14 in]
          }
          frame True {
            n124 = call "Master 10 kHz Reset.vi"("I/O Item"=w182) -> ("master 10 kHz reset"=w181:bool)  [unwired: 10 in]
          }
        }
      }
    }
    n125 = And(x="sync.counter reset enable", y=w39) -> (x .and. y?=w38:bool)
    n126 = feedback-in #11(w38) -> ()
    n127 = xnode "FPGA I/O Node"("I/O Item"=w67, "FPGA I/O In"=w65) -> ()  [unwired: 1 out]
    n128 = xnode "FPGA I/O Method Node"("FPGA I/O In"=w65, "Enable"="gain ranging.enable") -> ()  [unwired: 1 out]
    n129 = call <instrlib>:"Synchronous Latch.vi"("clear"="aurora.fifo overflow clear", "set"=w104) -> ("out"=→"aurora.fifo 1 overflow":bool)  [unwired: 9 in]
    n130 = call <instrlib>:"Synchronous Latch.vi"("clear"="aurora.fifo overflow clear", "set"=w100) -> ("out"=→"aurora.fifo 0 overflow":bool)  [unwired: 9 in]
    n131 = Unbundle By Name(w129) -> ("clear data in error"=w130:bool)
    n132 = call "Output Data.vi"("input data"=w56, "reset"=w35, "cal parameters"="cal.correction", "generation parameters"="cal.generation", "txjesd.clear data in error"=w130) -> ("txjesd.data in error"=w128:bool)  [unwired: 10 in]
    n133 = global write "Globals.vi" "data error"(w128) -> ()
  }
  n134 = timed-loop {
    timing: w12 -> [_]
    timing-out: [_] -> w11
    tunnel: w7 -> [w252]
    tunnel: w8 -> [w251]
    stop <- _ stop-if-true
    # "Single Port - 5.5GB/s"
    n135 = call "Aurora Reader (Single Port) .vi"("AXI4-Stream Reader FXP64x4"=w251) -> ("data"=w249:bool[], "output valid"=w248:bool)  [unwired: 13 in]
    n136 = case shown="True" w248 {
      tunnel: w249 -> [_ w259]
      tunnel: [FALSE ("Timed Out?") w258] -> w247
      frame False {
      }
      frame True {
        n137 = disable-structure shown="Disabled" {
          disable-tunnel: w259 -> [w262 _]
          disable-tunnel: [w260 _] -> w258
          frame Disabled {
            n138 = xnode ("FIFO Method Node")("Element"=w262, "Timeout"=0) -> ("Timed Out?"=w260:bool)  [unwired: 1 in, 1 out]
          }
          frame Enabled {
          }
        }
      }
    }
    n139 = call <instrlib>:"Synchronous Latch.vi"("clear"="port 4.rx fifo overflow clear", "set"=w247) -> ("out"=→"port 4.rx fifo overflow":bool)  [unwired: 9 in]
    n140 = call "Aurora Read Debug Signals (Single Port).vi"("Debug CLIP Resources"=T29 {"Hard Error"="7902R IO Socket\\uPort4_HardError", "Soft Error"="7902R IO Socket\\uPort4_SoftError", "Lane Up"="7902R IO Socket\\uPort4_LaneUp", "Channel Up"="7902R IO Socket\\uPort4_ChannelUp", "Sys Reset"="7902R IO Socket\\uPort4_sys_reset_out"}) -> ("Debug Info"=→"port 4.debug info":T2)  [unwired: 14 in]
    n141 = feedback #19(FALSE ("ready for input")) -> (w241:bool)
    n142 = case shown="True" w241 {
      tunnel: [_ w256] -> w250
      tunnel: [TRUE ("Timed Out?") w255] -> w244
      frame False {
      }
      frame True {
        n143 = xnode ("FIFO Method Node")("Timeout"=0) -> ("Element"=w256:bool[], "Timed Out?"=w255:bool)  [unwired: 1 in, 1 out]
      }
    }
    n144 = Not(x=w244) -> (.not. x?=w243:bool)
    n145 = call "Aurora Writer (Single Port).vi"("input data"=w250, "AXI4-Stream Writer FXP64x4"=w252, "input valid"=w243) -> ("ready for input"=w242:bool)  [unwired: 12 in]
    n146 = feedback-in #19(w242) -> ()
  }
  n147 = timed-loop {
    timing: w33 -> [_]
    timing-out: [_] -> w32
    stop <- _ stop-if-true
    # "CLIP Control and Status"
    n148 = Unbundle By Name("txjesd.control") -> ("reset"=w276:bool, "gtx enable"=w275:bool, "jesd enable"=w274:bool, "sw sync"=w273:bool, "gtx post cursor"=w272:fxp<+,5,5>, "gtx pre cursor"=w271:fxp<+,5,5>, "gtx diff control"=w270:fxp<+,4,4>, "clock enable"=w269:bool, "lmfc delay"=w268:fxp<+,5,5>)
    n149 = global write "Globals.vi" "txjesd.control"("txjesd.control") -> ()
    n150 = xnode "FPGA I/O Node"("7902R IO Socket\\aResetSl"=w276, "7902R IO Socket\\aGtxEnable"=w275, "7902R IO Socket\\aJesdEnable"=w274, "7902R IO Socket\\aSyncFromSw"=w273, "7902R IO Socket\\aGtxPostCursor"=w272, "7902R IO Socket\\aGtxPreCursor"=w271, "7902R IO Socket\\aGtxDiffCntrl"=w270, "7902R IO Socket\\aClkEnable"=w269, "7902R IO Socket\\aLmfcDly"=w268) -> ()  [unwired: 9 in, 9 out]
    n151 = xnode "FPGA I/O Node"() -> ("7902R IO Socket\\aGtxActive"=w286:bool, "7902R IO Socket\\aJesdActive"=w280:bool, "7902R IO Socket\\aLaneSyncReq"=w281:bool, "7902R IO Socket\\aLanesSynced"=w282:bool, "7902R IO Socket\\aLanesAligned"=w283:bool, "7902R IO Socket\\aQpllLocked"=w284:bool, "7902R IO Socket\\aQpllRefLost"=w285:bool, "7902R IO Socket\\MgtRefClks_Locked"=w278:bool, "7902R IO Socket\\MgtRefClks_Valid"=w277:bool)  [unwired: 9 in, 9 out]
    n152 = global read "Globals.vi" "data error"() -> (w265:bool)
    n153 = Bundle By Name(cluster=T9 {"gtx active"=FALSE, "jesd active"=FALSE, "lane sync req"=FALSE, "lanes synced"=FALSE, "lanes aligned"=FALSE, "qpll locked"=FALSE, "qpll ref lost"=FALSE, "mgt ref clocks locked"=FALSE, "mgt ref clock valid"=FALSE, "data error"=FALSE} ("txjesd.status 2"), "gtx active"=w286, "jesd active"=w280, "lane sync req"=w281, "lanes synced"=w282, "lanes aligned"=w283, "qpll locked"=w284, "qpll ref lost"=w285, "mgt ref clocks locked"=w278, "mgt ref clock valid"=w277, "data error"=w265) -> (→"txjesd.status":T9)
  }
  n154 = node-c288(w11) -> ()
  n155 = node-c288 ("Input Node")() -> (w10:T22)  [unwired: 1 in]
  n156 = call "Aurora Create Resources (Single Port).vi"("RX CLIP Resources"=T20 {"m_axis_tvalid"="7902R IO Socket\\uPort5_m_axi_rx_tvalid", "m_axis_tdata_0"="7902R IO Socket\\uPort5_m_axi_rx_tdata_0", "m_axis_tdata_1"="7902R IO Socket\\uPort5_m_axi_rx_tdata_1", "m_axis_tdata_2"="7902R IO Socket\\uPort5_m_axi_rx_tdata_2", "m_axis_tdata_3"="7902R IO Socket\\uPort5_m_axi_rx_tdata_3"}, "TX CLIP Resources"=T19 {"s_axis_tvalid"="7902R IO Socket\\uPort5_s_axi_tx_tvalid", "s_axis_tdata_0"="7902R IO Socket\\uPort5_s_axi_tx_tdata_0", "s_axis_tdata_1"="7902R IO Socket\\uPort5_s_axi_tx_tdata_1", "s_axis_tdata_2"="7902R IO Socket\\uPort5_s_axi_tx_tdata_2", "s_axis_tdata_3"="7902R IO Socket\\uPort5_s_axi_tx_tdata_3", "s_axis_tready"="7902R IO Socket\\uPort5_s_axi_tx_tready"}) -> ("AXI4-Stream Reader FXP64x4"=w4:T25, "AXI4-Stream Writer FXP64x4"=w3:T26)  [unwired: 8 in]
  n157 = node-c288(w32) -> ()
  n158 = timed-loop {
    timing: w10 -> [_]
    timing-out: [_] -> w9
    tunnel: w3 -> [w289]
    tunnel: w4 -> [w293]
    stop <- _ stop-if-true
    # "Single Port - 5.5GB/s"
    n159 = call "Aurora Reader (Single Port) .vi"("AXI4-Stream Reader FXP64x4"=w293) -> ("data"=w295:bool[], "output valid"=w294:bool)  [unwired: 13 in]
    n160 = case shown="True" w294 {
      tunnel: w295 -> [_ w310]
      tunnel: [FALSE ("Timed Out?") w309] -> w301
      frame False {
      }
      frame True {
        n161 = disable-structure shown="Disabled" {
          disable-tunnel: w310 -> [w313 _]
          disable-tunnel: [w311 _] -> w309
          frame Disabled {
            n162 = xnode ("FIFO Method Node")("Element"=w313, "Timeout"=0) -> ("Timed Out?"=w311:bool)  [unwired: 1 in, 1 out]
          }
          frame Enabled {
          }
        }
      }
    }
    n163 = call <instrlib>:"Synchronous Latch.vi"("clear"="port 5.rx fifo overflow clear", "set"=w301) -> ("out"=→"port 5.rx fifo overflow":bool)  [unwired: 9 in]
    n164 = call "Aurora Read Debug Signals (Single Port).vi"("Debug CLIP Resources"=T29 {"Hard Error"="7902R IO Socket\\uPort5_HardError", "Soft Error"="7902R IO Socket\\uPort5_SoftError", "Lane Up"="7902R IO Socket\\uPort5_LaneUp", "Channel Up"="7902R IO Socket\\uPort5_ChannelUp", "Sys Reset"="7902R IO Socket\\uPort5_sys_reset_out"}) -> ("Debug Info"=→"port 5.debug info":T2)  [unwired: 14 in]
    n165 = feedback #20(FALSE ("ready for input")) -> (w297:bool)
    n166 = case shown="True" w297 {
      tunnel: [_ w307] -> w292
      tunnel: [TRUE ("Timed Out?") w306] -> w298
      frame False {
      }
      frame True {
        n167 = xnode ("FIFO Method Node")("Timeout"=0) -> ("Element"=w307:bool[], "Timed Out?"=w306:bool)  [unwired: 1 in, 1 out]
      }
    }
    n168 = Not(x=w298) -> (.not. x?=w291:bool)
    n169 = call "Aurora Writer (Single Port).vi"("input data"=w292, "AXI4-Stream Writer FXP64x4"=w289, "input valid"=w291) -> ("ready for input"=w290:bool)  [unwired: 12 in]
    n170 = feedback-in #20(w290) -> ()
  }
  n171 = xnode "VI-Defined Handshake"() -> ("Handshake Out"=w25:refnum<k21>)
  n172 = xnode "VI-Defined Handshake"() -> ("Handshake Out"=w24:refnum<k21>)
  n173 = xnode "VI-Defined Handshake"() -> ("Handshake Out"=w22:refnum<k21>)
  n174 = xnode "VI-Defined Handshake"() -> ("Handshake Out"=w18:refnum<k21>)
  n175 = xnode "VI-Defined Handshake"() -> ("Handshake Out"=w19:refnum<k21>)
  n176 = xnode "VI-Defined Handshake"() -> ("Handshake Out"=w16:refnum<k21>)
  n177 = xnode "VI-Defined Handshake"() -> ("Handshake Out"=w15:refnum<k21>)
  n178 = node-c288() -> (w28:T22)  [unwired: 1 in]
  n179 = call "Monitor Clock Process.vi"("clock name"=refnum<k21> "40 MHz Onboard Clock", "handshake"=w25) -> ()  [unwired: 14 in]
  n180 = call "Monitor Clock Process.vi"("clock name"=refnum<k21> "100 MHz Clock", "handshake"=w24) -> ()  [unwired: 14 in]
  n181 = call "Monitor Clock Process.vi"("clock name"=refnum<k21> "7902R IO Socket\\SampleClk", "handshake"=w22) -> ()  [unwired: 14 in]
  n182 = call "Monitor Clock Process.vi"("clock name"=refnum<k21> "7902R IO Socket\\SampleClkx2", "handshake"=w18) -> ()  [unwired: 14 in]
  n183 = call "Monitor Clock Process.vi"("clock name"=refnum<k21> "7902R IO Socket\\SampleClkDiv2", "handshake"=w19) -> ()  [unwired: 14 in]
  n184 = call "Monitor Clock Process.vi"("clock name"=refnum<k21> "7902R IO Socket\\Port4_UserClk", "handshake"=w16) -> ()  [unwired: 14 in]
  n185 = call "Monitor Clock Process.vi"("clock name"=refnum<k21> "7902R IO Socket\\Port5_UserClk", "handshake"=w15) -> ()  [unwired: 14 in]
  n186 = timed-loop {
    timing: w28 -> [_]
    timing-out: [_] -> w27
    tunnel: w25 -> [w330]
    tunnel: w24 -> [w329]
    tunnel: w22 -> [w325]
    tunnel: w18 -> [w322]
    tunnel: w19 -> [w323]
    tunnel: w16 -> [w319]
    tunnel: w15 -> [w318]
    stop <- _ stop-if-true
    n187 = call "Get Clock State.vi"("handshake in"=w330) -> ("clock valid"=w328:bool)  [unwired: 14 in]
    n188 = call "Get Clock State.vi"("handshake in"=w329) -> ("clock valid"=w327:bool)  [unwired: 14 in]
    n189 = call "Get Clock State.vi"("handshake in"=w325) -> ("clock valid"=w324:bool)  [unwired: 14 in]
    n190 = call "Get Clock State.vi"("handshake in"=w322) -> ("clock valid"=w321:bool)  [unwired: 14 in]
    n191 = call "Get Clock State.vi"("handshake in"=w323) -> ("clock valid"=w320:bool)  [unwired: 14 in]
    n192 = call "Get Clock State.vi"("handshake in"=w319) -> ("clock valid"=w317:bool)  [unwired: 14 in]
    n193 = call "Get Clock State.vi"("handshake in"=w318) -> ("clock valid"=w316:bool)  [unwired: 14 in]
    n194 = Build Array(w328, w327, w324, w321, w320, w317, w316) -> (→"clocks valid":bool[])
  }
  n195 = node-c288(w27) -> ()
  n196 = node-c288(w9) -> ()
  n197 = node-c288(w30) -> ()
